vi "West Window Control.vi"(1 "Desired Window Open %":dbl) -> (0 "Error string":string)   [LabVIEW 2017]
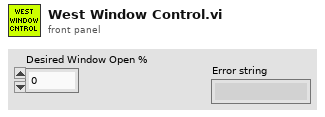
[diagram p1: front panel]
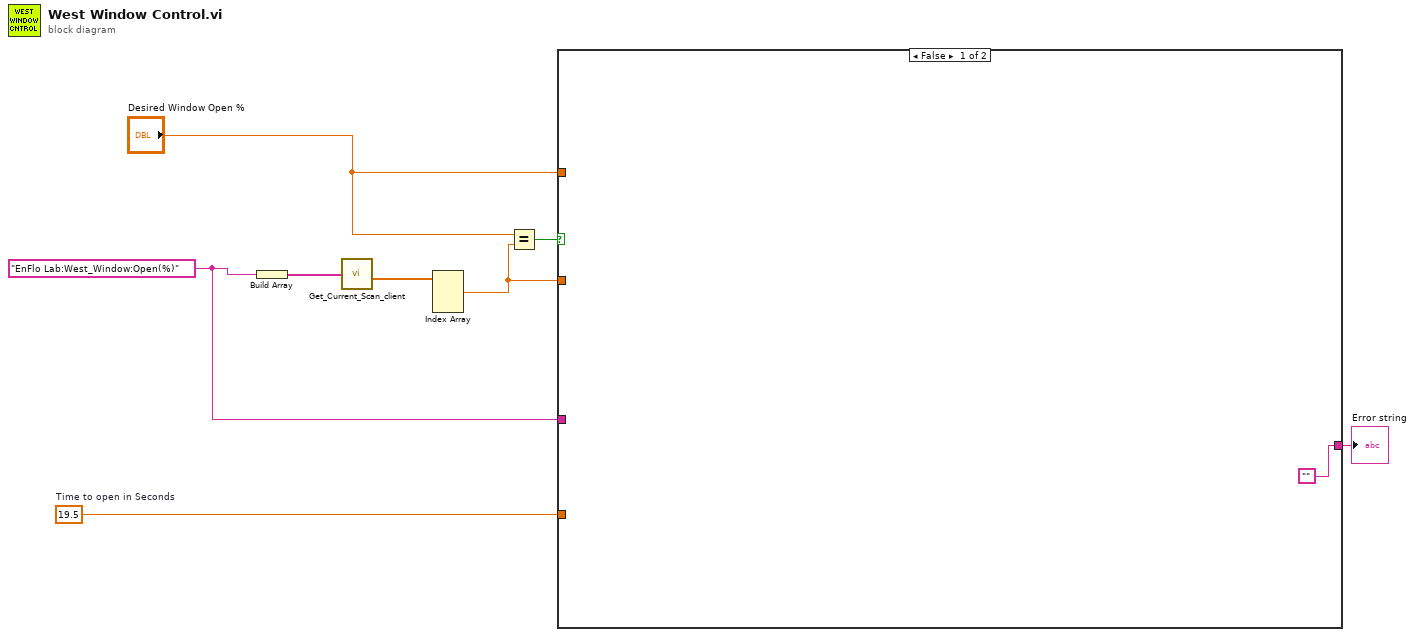
[diagram p0: block diagram]
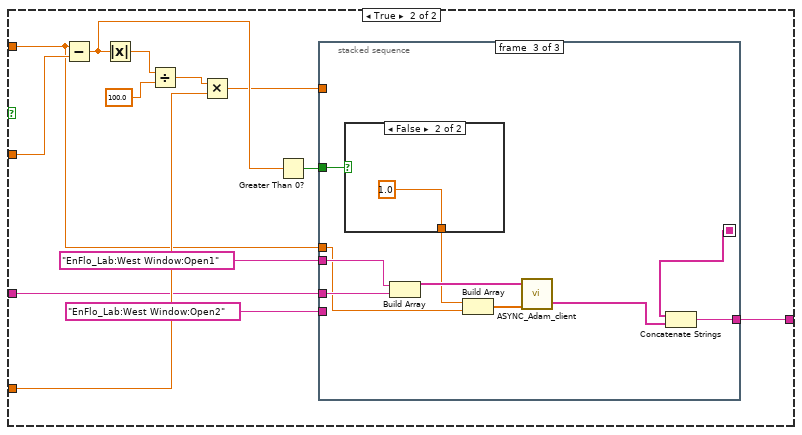
[diagram p2: hidden frame]
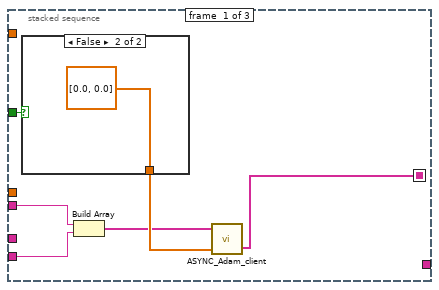
[diagram p3: hidden frame]
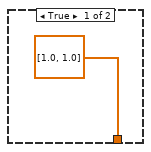
[diagram p4: hidden frame]
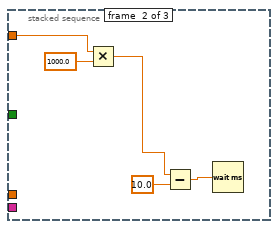
[diagram p5: hidden frame]
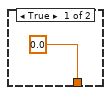
[diagram p6: hidden frame]
diagram:
  w3 = 19.5  # Time to open in Seconds
  w2 = "EnFlo Lab:West_Window:Open(%)"
  n1 = Build Array(w2) -> (w8:string[])
  n2 = call "Get_Current_Scan_client.vi"("ADAM Ch Names"=w8) -> ("Numerical Values"=w7:dbl[])  [unwired: 1 in, 2 out]
  n3 = Index Array(array=w7) -> (element #1=w4:dbl)  [unwired: 3 in, 2 out]
  n4 = Equal?(x="Desired Window Open %", y=w4) -> (x = y?=w6:bool)
  n5 = case shown="False" w6 {
    tunnel: "Desired Window Open %" -> [_ w11]
    tunnel: w4 -> [_ w22]
    tunnel: w3 -> [_ w19]
    tunnel: w2 -> [_ w12]
    tunnel: ["" w10] -> w1
    frame False {
    }
    frame True {
      n6 = Subtract(x=w11, y=w22) -> (x-y=w17:dbl)
      n7 = Absolute Value(x=w17) -> (abs(x)=w18:dbl)
      n8 = Divide(x=w18, y=100.0) -> (x/y=w20:dbl)
      n9 = Multiply(x=w20, y=w19) -> (x*y=w15:dbl)
      n10 = Greater Than 0?(x=w17) -> (x > 0?=w16:bool)
      n11 = stacked-sequence {
        seq-local: [w23 _ _] -> [_ _ w38]
        tunnel: w16 -> [w28 _ w45]
        tunnel: w15 -> [_ w35 _]
        tunnel: "EnFlo_Lab:West Window:Open1" -> [w26 _ w44]
        tunnel: "EnFlo_Lab:West Window:Open2" -> [w25 _ _]
        tunnel: w12 -> [_ _ w41]
        tunnel: w11 -> [_ _ w40]
        tunnel: [_ _ w36] -> w10
        frame #0 {
          n12 = case shown="False" w28 {
            tunnel: [dbl[] [1.0, 1.0] ("Values") dbl[] [0.0, 0.0] ("Values")] -> w27
            frame True {
            }
            frame False {
            }
          }
          n13 = Build Array(w26, w25) -> (w24:string[])
          n14 = call "ASYNC_Adam_client.vi"("Values"=w27, "Channel Names"=w24) -> ("Scan Comments"=w23:string[])  [unwired: 1 in, 1 out]
        }
        frame #1 {
          n15 = Multiply(x=w35, y=1000.0) -> (x*y=w33:dbl)
          n16 = Subtract(x=w33, y=10.0) -> (x-y=w31:dbl)
          n17 = Wait (ms)(milliseconds to wait=w31) -> ()  [unwired: 1 out]
        }
        frame #2 {
          n18 = case shown="False" w45 {
            tunnel: [0.0 1.0] -> w42
            frame True {
            }
            frame False {
            }
          }
          n19 = Build Array(w44, w41) -> (w43:string[])
          n20 = Build Array(w42, w40) -> (w39:dbl[])
          n21 = call "ASYNC_Adam_client.vi"("Values"=w39, "Channel Names"=w43) -> ("Scan Comments"=w37:string[])  [unwired: 1 in, 1 out]
          n22 = Concatenate Strings(w38, w37) -> (w36:string)
        }
      }
    }
  }
  "Error string" <- w1
